vi "sampling_frequency.vi"(9 "SF [Hz]":dbl, 11 "Connection":cluster{"queue out":refnum<queue>}) -> (3 "Connection 2":cluster{"queue out":refnum<queue>})   [LabVIEW 2019]
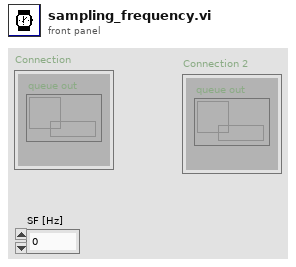
[diagram p1: front panel]
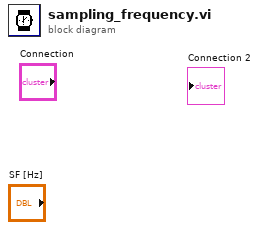
[diagram p0: block diagram]
diagram:
